vi "define.vi"(8 "error in (no error)":errorcluster, 11 "TrajectoryMG100122AODFrameScan in":refnum<class "TrajectoryMG100122AODFrameScan.lvclass">) -> (0 "error out":errorcluster, 3 "TrajectoryMG100122AODFrameScan out":refnum<class "TrajectoryMG100122AODFrameScan.lvclass">)   [LabVIEW 2010]
uses:
  common/classes/ImageCollection/ImageCollection/ImageCollection.lvclass
  common/classes/Image/Image/Image.lvclass
  fpga_VIs/FPGAMG100125AOD/FPGAMG100125AODFrameScan/FPGAMG100125AODFrameScan.lvclass
  FPGAWrapper/GenericFPGAWrapper/GenericFPGAWrapper/GenericFPGAWrapper.lvclass
  TrajectoryMG100122AODFrameScan.lvclass
panel:
  out "path out":path
  in  "power distribution":enum16{"constant", "linear", "exponential"}(ring)
  in  "reset":bool
  in  "accept":bool
  in  "load image":bool
  in  "Power":cluster{dbl, dbl}(slide)={100.00000000000004, 100.00000000000004} scale=1.0..100.0
  in  "Depth":dbl[unit](slide) min=0.0 step=1e-06
  out "Boolean":bool
  out "number of frames":i32
  out "Reference Image":T1(plugin-control)
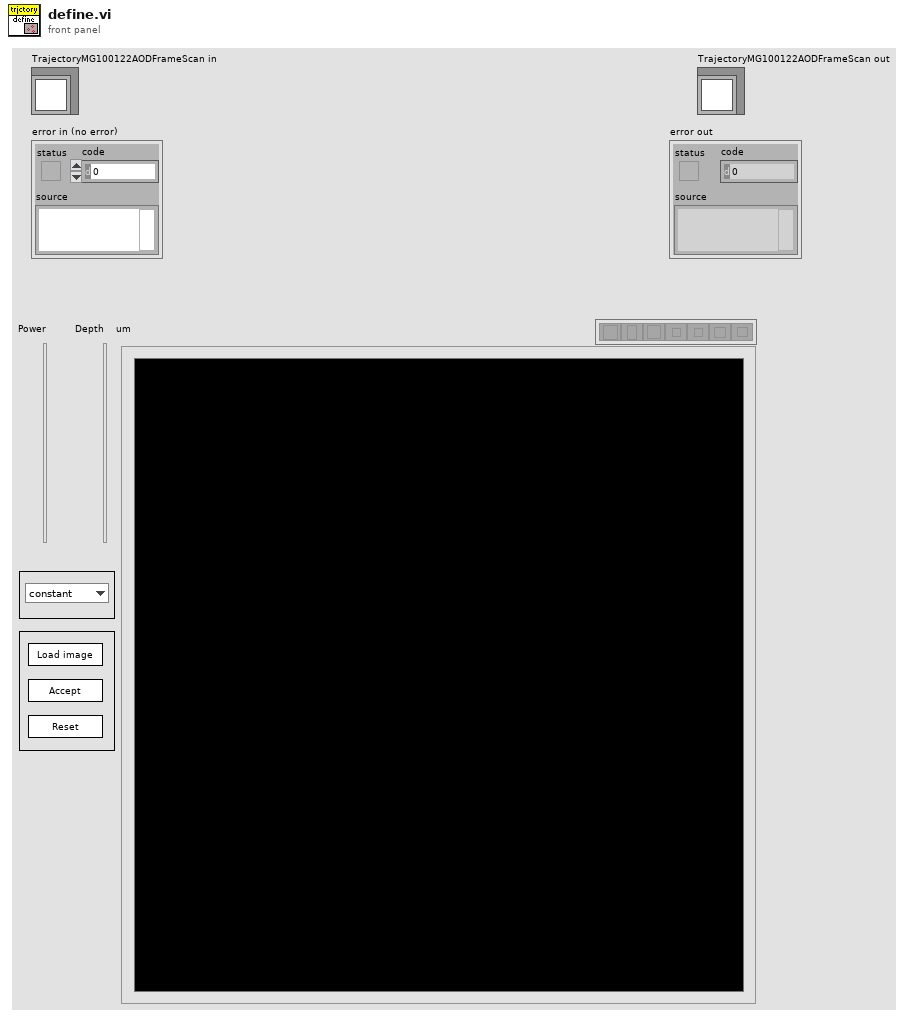
[diagram p1: front panel]
types:
  T1 = typedef "IMAQ Image.ctl" = refnum<image>
  T2 = cluster{"Global Rectangle":i32[], "Contours":cluster{"Contour Type":u32, "ROI Type":u32, "Points":i32[]}[]}
  T3 = cluster{"Global Rectangle":i32[], "Contours":cluster{"Contour Type":u32, "ROI Type":u32, "Points":i32[]}[]}[]
  T4 = typedef "Image Type" = u32
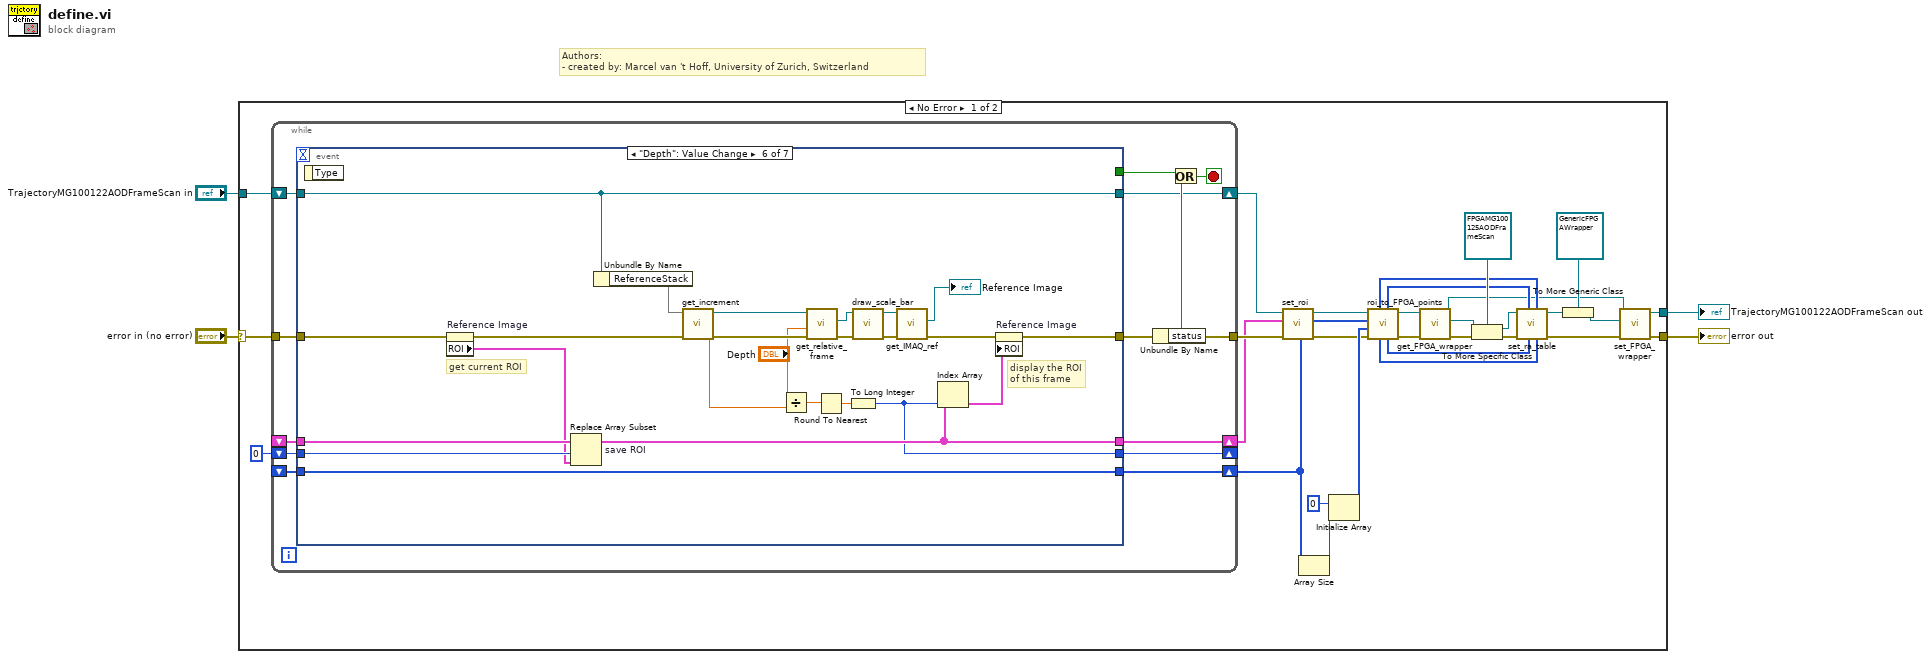
[diagram p0: block diagram]
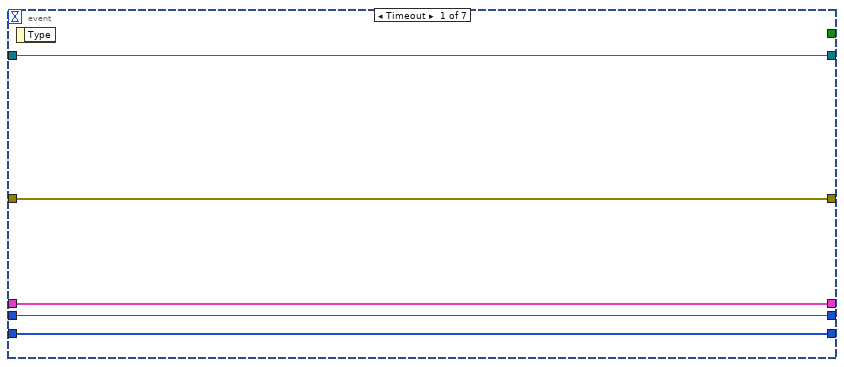
[diagram p2: hidden frame]
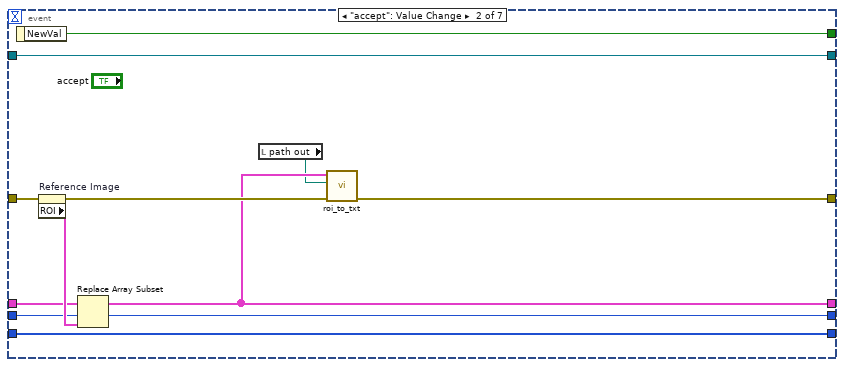
[diagram p3: hidden frame]
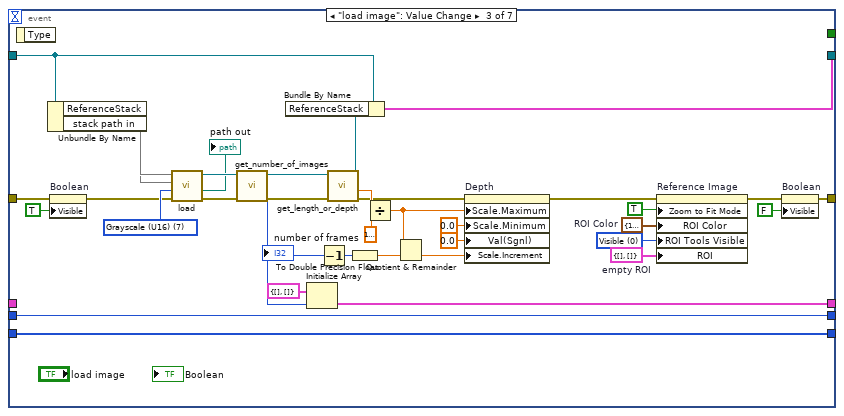
[diagram p4: hidden frame]
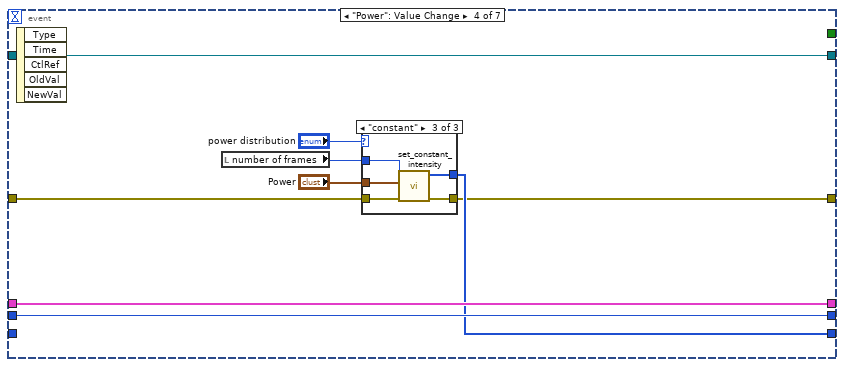
[diagram p5: hidden frame]
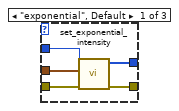
[diagram p6: hidden frame]
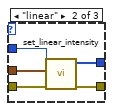
[diagram p7: hidden frame]
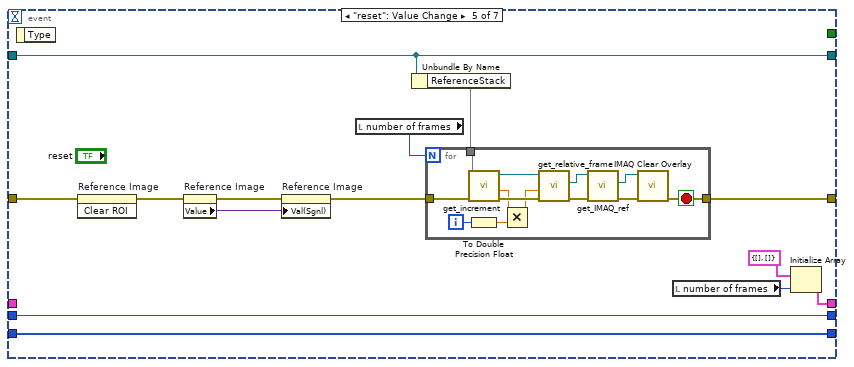
[diagram p8: hidden frame]
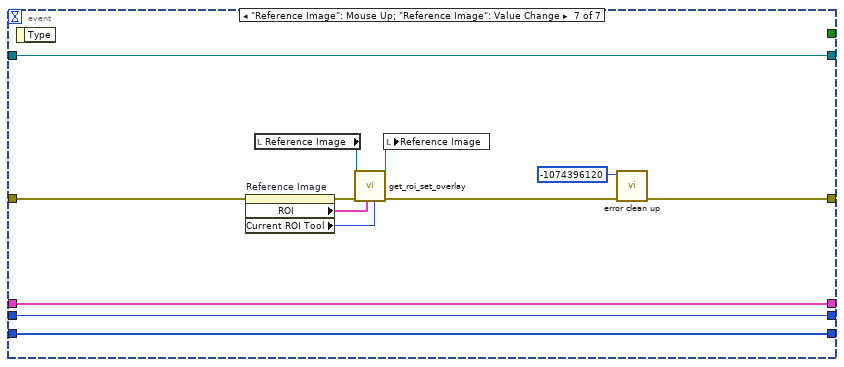
[diagram p9: hidden frame]
diagram:
  # "Authors: \n- created by: Marcel van 't Hoff, University of Zurich, Switzerland"
  n1 = case shown="No Error" "error in (no error)" {
    selector: "error in (no error)" -> [w34 w189]
    tunnel: [w15 w189] -> w3
    tunnel: [w17 w188] -> w1
    tunnel: "TrajectoryMG100122AODFrameScan in" -> [w32 w188]
    frame No Error {
      n2 = while {
        tunnel: w34 -> [w46]
        tunnel: [w45] -> w9
        shift-right: [w35] -> w8
        shift-left: w32 -> [w47]
        shift-right: [w38] -> w7
        shift-left: _ -> [w41]
        shift-right: [w40] -> _
        shift-left: 0 ("z-stack position") -> [w39]
        shift-right: [w37] -> w14
        shift-left: _ -> [w36]
        stop <- w42 stop-if-true
        n3 = event shown="[5] \"Depth\": Value Change" {
          selector: _ -> [_ _ _ _ _ _ _]
          dyn-events: _ -> [_ _ _ _ _ _ _]
          timeout: _ -> [_ _ _ _ _ _ _]
          tunnel: [_ w62 _ _ _ _ _] -> w44
          tunnel: w47 -> [w51 w63 w93 w108 w127 w170 w186]
          tunnel: w46 -> [w52 w61 w72 w102 w134 w166 w187]
          tunnel: [w52 w55 w68 w101 w128 w168 w176] -> w45
          tunnel: [w51 w63 w92 w108 w127 w170 w186] -> w35
          tunnel: [w50 w54 w80 w107 w135 w162 w179] -> w38
          tunnel: w41 -> [w50 w59 _ w107 _ w169 w179]
          tunnel: [w49 w58 w82 w106 w137 w153 w181] -> w40
          tunnel: w39 -> [w49 w58 w82 w106 w137 w167 w181]
          tunnel: [w48 w57 w66 w103 w124 w152 w178] -> w37
          tunnel: w36 -> [w48 w57 w66 _ w124 w152 w178]
          event Timeout {
            n4 = event-data() -> ()  [unwired: 1 in, 1 out]
          }
          event "accept": Value Change {
            n5 = event-data() -> ("NewVal"=w62:bool)  [unwired: 1 in]
            n6 = property on="Reference Image" class="ImageControl"(error in=w61) -> (error out=w56:errorcluster, "ROI"=w60:T2)  [unwired: 1 in, 1 out]
            n7 = Replace Array Subset(array=w59, new element=w60, index=w58) -> (w54:T3)
            n8 = local read "path out"() -> (w53:path)
            n9 = call "roi_to_txt.vi"("error in"=w56, "path in"=w53, "output array in"=w54) -> ("error out"=w55:errorcluster)  [unwired: 7 in, 1 out]
          }
          event "load image": Value Change {
            w79 = T2 {"Global Rectangle"=[], "Contours"=[]}  # empty ROI
            w83 = u32 0 items=["Visible", "Hidden", "Hidden, Use WindTools Palette"] ("ROI Tools Visible")
            w84 = cluster{"Red":u8, "Green":u8, "Blue":u8} {"Red"=100, "Green"=255, "Blue"=0}  # ROI Color
            w98 = T4 7 items=["Grayscale (U8)", "Grayscale (I16)", "Grayscale (SGL)", "Complex (CSG)", "RGB (U32)", "HSL (U32)", "RGB (U64)", "Grayscale (U16)"] ("Image Type")
            n10 = event-data() -> ()  [unwired: 1 in, 1 out]
            n11 = Unbundle By Name(w93) -> ("ReferenceStack"=w99, "stack path in"=w65)
            n12 = property on="Boolean" class="Bool (strict)"(error in=w72, "Visible"=TRUE) -> (error out=w71:errorcluster)  [unwired: 1 in, 1 out]
            n13 = call "load.vi"("error in (no error)"=w71, "Image Type"=w98, "path in"=w65, "ImageCollection in"=w99) -> ("error out"=w75:errorcluster, "path out"=→"path out":path, "ImageCollection out"=w77:refnum<class "ImageCollection.lvclass">)  [unwired: 3 in, 2 out]
            n14 = call-dynamic "get_number_of_images.vi"("error in (no error)"=w75, "ImageCollection in"=w77) -> ("error out"=w74:errorcluster, "size"=w73:i32, "ImageCollection out"=w76:refnum<class "ImageCollection.lvclass">)  [unwired: 7 in]
            "number of frames" <- w73
            n15 = Initialize Array(T2 {"Global Rectangle"=[], "Contours"=[]} ("ROI"), w73) -> (w80:T3)
            n16 = Decrement(x=w73) -> (x-1=w90:i32)
            n17 = call "get_length_or_depth.vi"("error in (no error)"=w74, "ImageCollection in"=w76) -> ("error out"=w78:errorcluster, "total z depth"=w96:dbl[unit], "ImageCollection out"=w91:refnum<class "ImageCollection.lvclass">)  [unwired: 5 in, 2 out]
            n18 = Bundle By Name(cluster=w93, "ReferenceStack"=w91) -> (w92:cluster{})
            n19 = To Double Precision Float(number=w90) -> (double precision float=w87:dbl)
            n20 = Divide(x=w96, y=dbl[unit] 1e-06) -> (x/y=w89:dbl)
            n21 = Quotient & Remainder(x=w89, y=w87) -> (floor(x/y)=w88:dbl)  [unwired: 1 out]
            n22 = property on="Depth" class="Slide (strict)"(error in=w78, "Scale.Maximum"=w89, "Scale.Minimum"=0.0 ("Scale.Range:Minimum"), "Val(Sgnl)"=dbl[unit] 0.0 ("y"), "Scale.Increment"=w88) -> (error out=w86:errorcluster)  [unwired: 1 in, 1 out]
            n23 = property on="Reference Image" class="ImageControl"(error in=w86, "Zoom to Fit Mode"=TRUE, "ROI Color"=w84, "ROI Tools Visible"=w83, "ROI"=w79) -> (error out=w69:errorcluster)  [unwired: 1 in, 1 out]
            n24 = property on="Boolean" class="Bool (strict)"(error in=w69, "Visible"=FALSE) -> (error out=w68:errorcluster)  [unwired: 1 in, 1 out]
          }
          event "Power": Value Change {
            n25 = event-data() -> ()  [unwired: 1 in, 5 out]
            n26 = local read "number of frames"() -> (w104:i32)
            n27 = case shown="\"constant\"" "power distribution" {
              tunnel: "Power" -> [w109 w118 w119]
              tunnel: w104 -> [w110 w117 w120]
              tunnel: [w111 w116 w121] -> w103
              tunnel: w102 -> [w113 w115 w123]
              tunnel: [w112 w114 w122] -> w101
              frame "exponential", Default {
                n28 = call "set_exponential_intensity.vi"("error in (no error)"=w113, "power slider in"=w109, "number of frames"=w110) -> ("error out"=w112:errorcluster, "amplitude out"=w111:u16[])  [unwired: 7 in]
              }
              frame "linear" {
                n29 = call "set_linear_intensity.vi"("error in (no error)"=w115, "power slider in"=w118, "number of frames"=w117) -> ("error out"=w114:errorcluster, "amplitude out"=w116:u16[])  [unwired: 7 in]
              }
              frame "constant" {
                n30 = call "set_constant_intensity.vi"("error in (no error)"=w123, "power slider in"=w119, "number of frames"=w120) -> ("error out"=w122:errorcluster, "amplitude out"=w121:u16[])  [unwired: 7 in]
              }
            }
          }
          event "reset": Value Change {
            n31 = event-data() -> ()  [unwired: 1 in, 1 out]
            n32 = invoke on="Reference Image" class="ImageControl" method="Clear ROI"(error in=w134) -> (error out=w133:errorcluster)  [unwired: 2 in, 2 out]
            n33 = property on="Reference Image" class="ImageControl"(error in=w133) -> (error out=w132:errorcluster, "Value"=w131:variant)  [unwired: 1 in, 1 out]
            n34 = property on="Reference Image" class="ImageControl"(error in=w132, "Val(Sgnl)"=w131) -> (error out=w129:errorcluster)  [unwired: 1 in, 1 out]
            n35 = local read "number of frames"() -> (w125:i32)
            n36 = Unbundle By Name(w127) -> ("ReferenceStack"=w126)
            n37 = for {
              N: w125 -> [_]
              tunnel: [w146] -> w128
              tunnel: w129 -> [w143]
              tunnel: w126 -> [w145]
              i -> [w141]
              stop <- w146 stop-if-true
              n38 = call "get_increment.vi"("error in (no error)"=w143, "ImageCollection in"=w145) -> ("error out"=w142:errorcluster, "z increment"=w140:dbl[unit], "ImageCollection out"=w144:refnum<class "ImageCollection.lvclass">)  [unwired: 5 in, 2 out]
              n39 = To Double Precision Float(number=w141) -> (double precision float=w138:dbl)
              n40 = Multiply(x=w140, y=w138) -> (x*y=w139:dbl[unit])
              n41 = call-dynamic "get_relative_frame.vi"("error in (no error)"=w142, "relative depth"=w139, "ImageCollection in"=w144) -> ("error out"=w148:errorcluster, "frame"=w150:refnum<class "Image.lvclass">)  [unwired: 5 in, 2 out]
              n42 = call-dynamic "get_IMAQ_ref.vi"("error in (no error)"=w148, "Image.lvclass in"=w150) -> ("error out"=w147:errorcluster, "Image"=w149:T1)  [unwired: 5 in, 3 out]
              n43 = call "IMAQ Clear Overlay"("error in (no error)"=w147, "Image"=w149) -> ("error out"=w146:errorcluster)  [unwired: 8 in, 1 out]
            }
            n44 = local read "number of frames"() -> (w130:i32)
            n45 = Initialize Array(T2 {"Global Rectangle"=[], "Contours"=[]} ("ROI"), w130) -> (w135:T3)
          }
          event "Depth": Value Change {
            # "display the ROI\nof this frame"
            # "get current ROI"
            n46 = event-data() -> ()  [unwired: 1 in, 1 out]
            n47 = property on="Reference Image" class="ImageControl"(error in=w166) -> (error out=w154:errorcluster, "ROI"=w163:T2)  [unwired: 1 in, 1 out]
            n48 = Replace Array Subset "save ROI"(array=w169, new element=w163, index=w167) -> (w162:T3)
            n49 = Unbundle By Name(w170) -> ("ReferenceStack"=w155)
            n50 = call "get_increment.vi"("error in (no error)"=w154, "ImageCollection in"=w155) -> ("error out"=w160:errorcluster, "z increment"=w156:dbl[unit], "ImageCollection out"=w161:refnum<class "ImageCollection.lvclass">)  [unwired: 5 in, 2 out]
            n51 = Divide(x="Depth", y=w156) -> (x/y=w158:dbl)
            n52 = call-dynamic "get_relative_frame.vi"("error in (no error)"=w160, "relative depth"="Depth", "ImageCollection in"=w161) -> ("error out"=w173:errorcluster, "frame"=w172:refnum<class "Image.lvclass">)  [unwired: 5 in, 2 out]
            n53 = Round To Nearest(number=w158) -> (nearest integer value=w159:dbl)
            n54 = To Long Integer(number=w159) -> (32bit integer=w153:i32)
            n55 = call "draw_scale_bar.vi"("error in (no error)"=w173, "Image in"=w172) -> ("error out"=w174:errorcluster, "Image out"=w171:refnum<class "Image.lvclass">)  [unwired: 8 in]
            n56 = call-dynamic "get_IMAQ_ref.vi"("error in (no error)"=w174, "Image.lvclass in"=w171) -> ("error out"=w165:errorcluster, "Image"=→"Reference Image":T1)  [unwired: 5 in, 3 out]
            n57 = Index Array(array=w162, index=w153) -> (element=w164:T2)
            n58 = property on="Reference Image" class="ImageControl"(error in=w165, "ROI"=w164) -> (error out=w168:errorcluster)  [unwired: 1 in, 1 out]
          }
          event "Reference Image": Mouse Up; "Reference Image": Value Change {
            n59 = event-data() -> ()  [unwired: 1 in, 1 out]
            n60 = property on="Reference Image" class="ImageControl"(error in=w187) -> (error out=w185:errorcluster, "ROI"=w184:T2, "Current ROI Tool"=w183:u32)  [unwired: 1 in, 1 out]
            n61 = local read "Reference Image"() -> (w180:T1)
            n62 = call "get_roi_set_overlay.vi"("Current ROI Tool in"=w183, "ROI in"=w184, "error in"=w185, "Reference Image in"=w180) -> ("error out"=w177:errorcluster, "Reference Image out"=w182:T1)  [unwired: 6 in]
            n63 = local write "Reference Image"(w182) -> ()
            n64 = call <userlib>:"error clean up.vi"("error in"=w177, "code in"=-1074396120) -> ("error out"=w176:errorcluster)  [unwired: 9 in]
          }
        }
        n65 = Unbundle By Name(w45) -> ("status"=w43:bool)
        n66 = Or(x=w44, y=w43) -> (x .or. y?=w42:bool)
      }
      n67 = call-dynamic "set_roi.vi"("error in (no error)"=w9, "Array"=w7, "TrajectoryMG100122AODFrameScan in"=w8) -> ("error out"=w10:errorcluster, "TrajectoryMG100122AODFrameScan out"=w6:refnum<class "TrajectoryMG100122AODFrameScan.lvclass">)  [unwired: 7 in]
      n68 = Array Size(array=w14) -> (size(s)=w13:i32)
      n69 = Initialize Array(u16 0 ("element"), w13) -> (w11:u16[])
      n70 = call-dynamic "roi_to_FPGA_points.vi"("error in"=w10, "z in"=w11, "amplitude in"=w14, "TrajectoryMG100122AODFrameScan in"=w6) -> ("error out"=w27:errorcluster, "TrajectoryMG100122AODFrameScan out"=w5:refnum<class "TrajectoryMG100122AODFrameScan.lvclass">, "z out"=w23:u16[], "y out"=w24:u16[], "amp out"=w22:u16[], "x out"=w25:u16[])  [unwired: 2 in]
      n71 = call-dynamic "get_FPGA_wrapper.vi"("error in (no error)"=w27, "TrajectoryMG100122GenericFPGA in"=w5) -> ("error out"=w28:errorcluster, "GenericFPGAWrapper.lvclass"=w31:refnum<class "GenericFPGAWrapper.lvclass">, "TrajectoryMG100122GenericFPGA out"=w18:refnum<class "TrajectoryMG100122AODFrameScan.lvclass">)  [unwired: 7 in]
      n72 = To More Specific Class(target class=refnum<class "FPGAMG100125AODFrameScan.lvclass"> refnum ("FPGAMG100125AODFrameScan.lvclass"), reference=w31, error in=w28) -> (specific class reference=w30:refnum<class "FPGAMG100125AODFrameScan.lvclass">, error out=w26:errorcluster)
      n73 = call-dynamic "set_ra_table.vi"("amp"=w22, "x"=w25, "z"=w23, "y"=w24, "error in (no error)"=w26, "FPGAMG100125AODFrameScan in"=w30) -> ("error out"=w16:errorcluster, "FPGAMG100125AODFrameScan out"=w21:refnum<class "FPGAMG100125AODFrameScan.lvclass">)  [unwired: 3 in, 1 out]
      n74 = To More Generic Class(target class=refnum<class "GenericFPGAWrapper.lvclass"> refnum ("GenericFPGAWrapper.lvclass"), reference=w21) -> (generic class reference=w19:refnum<class "GenericFPGAWrapper.lvclass">)
      n75 = call-dynamic "set_FPGA_wrapper.vi"("error in (no error)"=w16, "GenericFPGAWrapper.lvclass"=w19, "TrajectoryMG100122GenericFPGA in"=w18) -> ("error out"=w15:errorcluster, "TrajectoryMG100122GenericFPGA out"=w17:refnum<class "TrajectoryMG100122AODFrameScan.lvclass">)  [unwired: 7 in]
    }
    frame Error {
    }
  }
  "error out" <- w3
  "TrajectoryMG100122AODFrameScan out" <- w1
